vi "SetError.vi"(7 "布尔":bool, 9 "错误输入（无错误）":errorcluster, 10 "CH":string) -> (1 "错误输出":errorcluster)   [LabVIEW 2013]
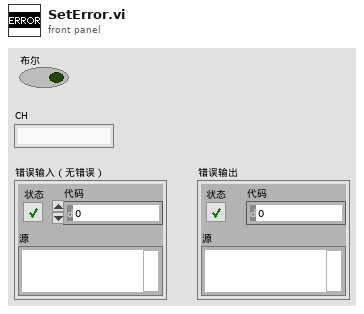
[diagram p1: front panel]
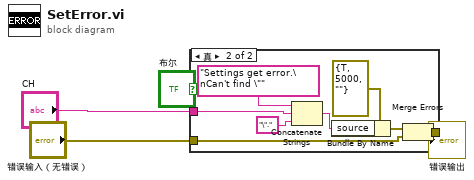
[diagram p0: block diagram]
diagram:
  n1 = case shown="真" "布尔" {
    tunnel: "错误输入（无错误）" -> [w5 w9]
    tunnel: [w5 w8] -> w3
    tunnel: "CH" -> [_ w7]
    frame False {
    }
    frame True {
      n2 = Concatenate Strings("Settings get error.\nCan't find \"" ("message"), w7, "\"." ("string")) -> (w12:string)
      n3 = Bundle By Name(cluster=errorcluster {"status"=TRUE, "code"=5000, "source"=""} ("error in 1 (no error)"), "source"=w12) -> (w11:errorcluster)
      n4 = Merge Errors(w11, w9) -> (w8:errorcluster)
    }
  }
  "错误输出" <- w3
